vi "CheckClick.vi"(6 "Enum":enum16{"MouseClick", "DropDown"}(ring), 7 "Pad":string, 8 "error in (no error)":errorcluster, 10 "Coords":T1, 11 "EpiWrapper in":refnum<class "EpiWrapper.lvclass">) -> (0 "error out":errorcluster, 1 "OnPad?":bool, 2 "Selected?":bool, 3 "EpiWrapper out":refnum<class "EpiWrapper.lvclass">, 4 "Id":string)   [LabVIEW 2012, in "EpiWrapper.lvclass"]
uses:
  EpiWrapper.lvclass
  <vilib>/Utility/miscctls.llb/LVPoint32TypeDef.ctl
  EpiWrapper.lvclass/EpiWrapper.ctl
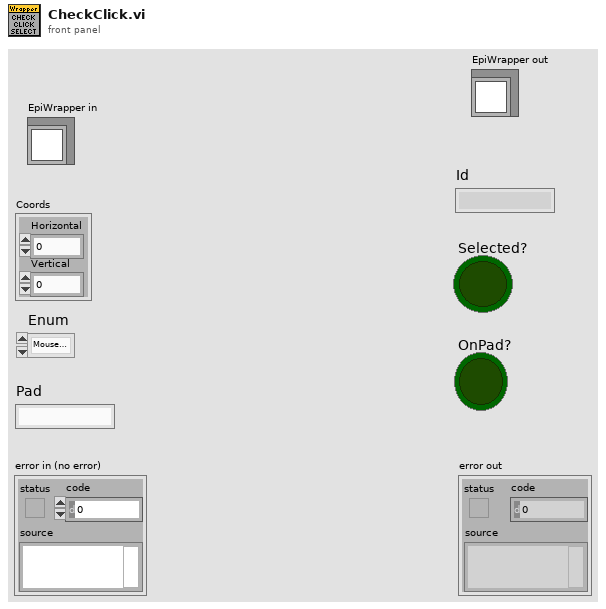
[diagram p1: front panel]
types:
  T1 = typedef "LVPoint32TypeDef.ctl" = cluster{"Horizontal":i32, "Vertical":i32}
  T2 = typedef "MapPOS.ctl" = cluster{"Coords":cluster{"Horizontal":sgl, "Vertical":sgl}, "radius":i32, "state":bool, "Id":string}[]
  T3 = typedef "SelectedPads.ctl" = T4[]
  T4 = typedef "Pad.ctl" = cluster{"Coords":cluster{"Horizontal":sgl, "Vertical":sgl}, "radius":i32, "Tested":bool, "Selected":bool, "Id":string}
  T5 = typedef "CurrentPad.ctl" = cluster{"Coords":cluster{"Horizontal":sgl, "Vertical":sgl}, "radius":i32, "Tested":bool, "Selected":bool, "Pad":string, "PadArea":T6}
  T6 = typedef "PadArea.ctl" = enum16{"A", "B", "C", "D", "L", "R", "T", "G"}
  T7 = typedef "MeasureControl.ctl" = cluster{"Graph":cluster{"Y":dbl[], "Y":dbl[]}[], "Pass":bool, "Fail":bool, "Measure":bool, "Wafer Area":T6, "TestData":T8, "Pad":string}
  T8 = typedef "TestData.ctl" = cluster{"20mA Data":T9, "50mA Data ":T9}
  T9 = typedef "Measurement.ctl" = cluster{"Area":string, "Pad":string, "Current,mA":dbl, "Power":dbl, "WL":dbl, "Voltage":dbl, "Knee Current":dbl, "Reverse":dbl}
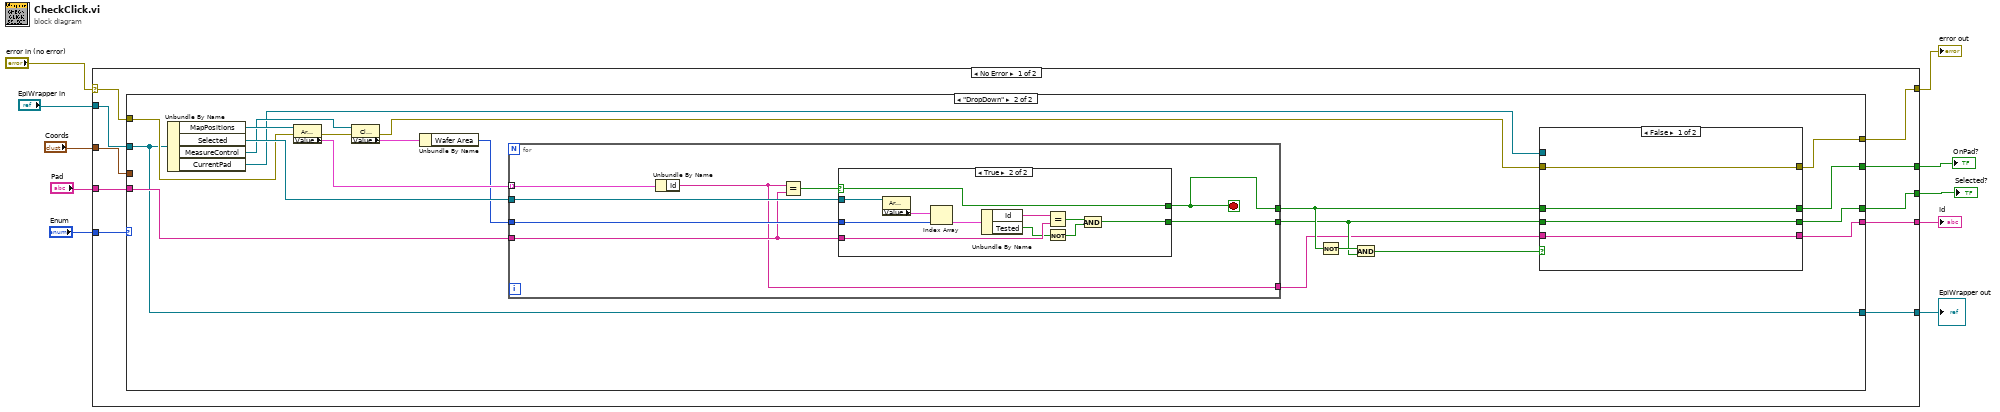
[diagram p0: block diagram]
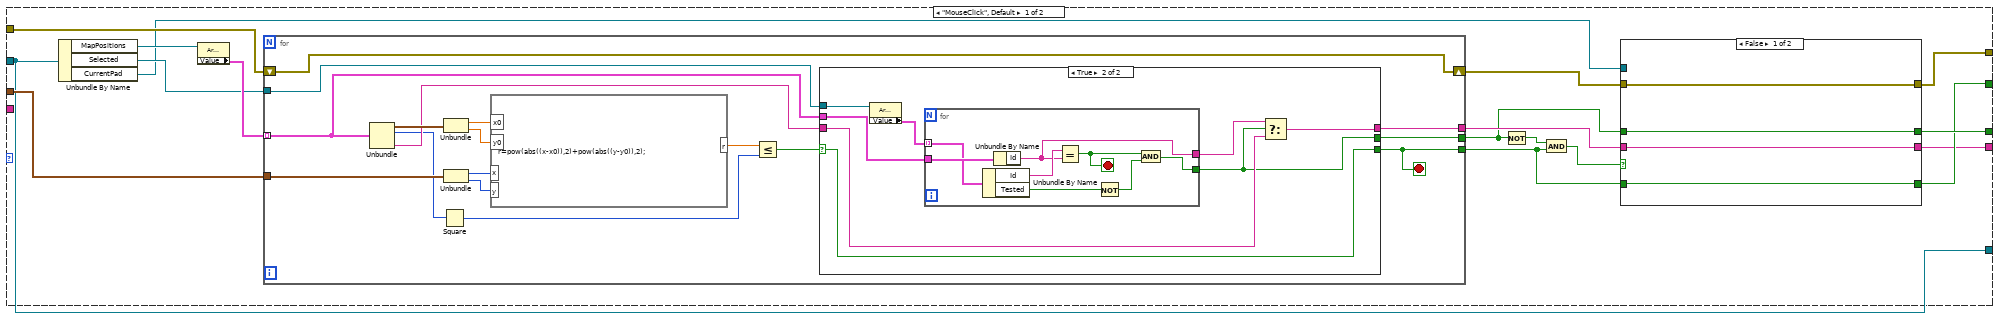
[diagram p2: hidden frame]
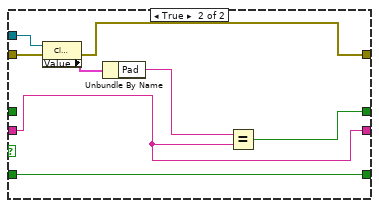
[diagram p3: hidden frame]
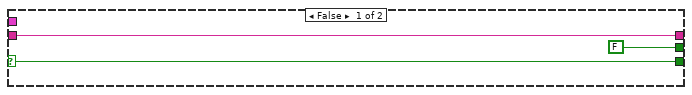
[diagram p4: hidden frame]
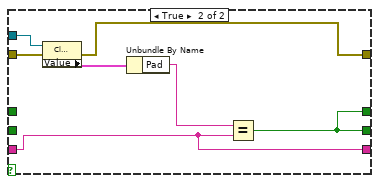
[diagram p5: hidden frame]
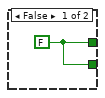
[diagram p6: hidden frame]
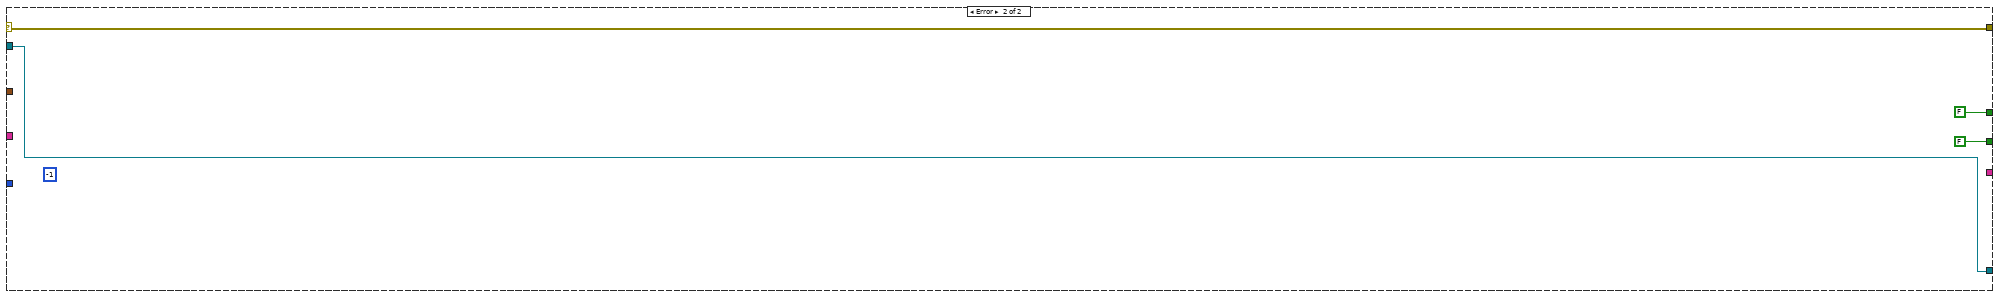
[diagram p7: hidden frame]
diagram:
  n1 = case shown="No Error" "error in (no error)" {
    selector: "error in (no error)" -> [w17 w141]
    tunnel: [w16 w141] -> w9
    tunnel: [w11 w140] -> w7
    tunnel: "EpiWrapper in" -> [w15 w140]
    tunnel: "Coords" -> [w20 _]
    tunnel: [w19 FALSE] -> w5
    tunnel: [w18 FALSE] -> w4
    tunnel: [w14 _] -> w3
    tunnel: "Enum" -> [w13 _]
    tunnel: "Pad" -> [w12 _]
    frame No Error {
      n2 = case shown="\"DropDown\"" w13 {
        tunnel: w20 -> [w35 _]
        tunnel: [w31 w92] -> w19
        tunnel: [w27 w91] -> w18
        tunnel: w17 -> [w33 w102]
        tunnel: [w23 w86] -> w16
        tunnel: w15 -> [w32 w99]
        tunnel: [w26 w88] -> w14
        tunnel: w12 -> [_ w104]
        tunnel: [w32 w99] -> w11
        frame "MouseClick", Default {
          n3 = Unbundle By Name(w32) -> ("MapPositions"=w37:refnum<vi>, "Selected"=w34:refnum<vi>, "CurrentPad"=w25:refnum<vi>)
          n4 = property class="Arr (strict)"(reference=w37) -> ("Value"=w36:T2)  [unwired: 1 in, 2 out]
          n5 = for {
            tunnel: w36 -> [w57] mode=indexing
            tunnel: w35 -> [w60]
            tunnel: w34 -> [w58]
            tunnel: [w56] -> w21
            tunnel: [w55] -> w22
            shift-right: [w54] -> w30
            shift-left: w33 -> [w54]
            tunnel: [w53] -> w24
            stop <- w55 stop-if-true
            n6 = Unbundle(w57) -> ("Coords"=w63:cluster{"Horizontal":sgl, "Vertical":sgl}, "radius"=w51:i32, "Id"=w52:string)  [unwired: 1 out]
            n7 = Square(x=w51) -> (x^2=w50:i32)
            n8 = Unbundle(w63) -> ("Horizontal"=w62:sgl, "Vertical"=w61:sgl)
            n9 = Unbundle(w60) -> ("Horizontal"=w66:i32, "Vertical"=w65:i32)
            n10 = formula code="r=pow(abs((x-x0)),2)+pow(abs((y-y0)),2);"("x0"=w62, "y0"=w61, "x"=w66, "y"=w65) -> ("r"=w64:dbl)
            n11 = Less Or Equal?(x=w64, y=w50) -> (x <= y?=w59:bool)
            n12 = case shown="True" w59 {
              selector: w59 -> [w69 w77]
              tunnel: [w69 w77] -> w55
              tunnel: w58 -> [_ w76]
              tunnel: w57 -> [_ w70]
              tunnel: [FALSE w72] -> w56
              tunnel: [w67 w73] -> w53
              tunnel: w52 -> [w67 w74]
              frame False {
              }
              frame True {
                n13 = property on="Property Node" class="Arr (strict)"(reference=w76) -> ("Value"=w71:T3)  [unwired: 1 in, 2 out]
                n14 = for {
                  tunnel: w70 -> [w83]
                  tunnel: [w81] -> w72
                  tunnel: [w84] -> w75
                  tunnel: w71 -> [w82] mode=indexing
                  stop <- w78 stop-if-true
                  n15 = Unbundle By Name(w82) -> ("Id"=w85:string, "Tested"=w80:bool)
                  n16 = Unbundle By Name(w83) -> ("Id"=w84:string)
                  n17 = Equal?(x=w85, y=w84) -> (x = y?=w78:bool)
                  n18 = Not(x=w80) -> (.not. x?=w79:bool)
                  n19 = And(x=w78, y=w79) -> (x .and. y?=w81:bool)
                }
                n20 = Select(t=w75, s=w72, f=w74) -> (s? t:f=w73:string)
              }
            }
          }
          n21 = Not(x=w21) -> (.not. x?=w28:bool)
          n22 = And(x=w28, y=w22) -> (x .and. y?=w29:bool)
          n23 = case shown="False" w29 {
            tunnel: [w39 w45] -> w31
            tunnel: w25 -> [_ w49]
            tunnel: w30 -> [w38 w48]
            tunnel: [w41 w44] -> w27
            tunnel: [w40 w42] -> w26
            tunnel: w22 -> [w41 w44]
            tunnel: w24 -> [w40 w42]
            tunnel: w21 -> [w39 _]
            tunnel: [w38 w46] -> w23
            frame False {
            }
            frame True {
              n24 = property class="Clust (strict)"(reference=w49, error in=w48) -> (error out=w46:errorcluster, "Value"=w47:T5)  [unwired: 1 out]
              n25 = Unbundle By Name(w47) -> ("Pad"=w43:string)
              n26 = Equal?(x=w43, y=w42) -> (x = y?=w45:bool)
            }
          }
        }
        frame "DropDown" {
          n27 = Unbundle By Name(w99) -> ("MapPositions"=w106:refnum<vi>, "Selected"=w103:refnum<vi>, "MeasureControl"=w101:refnum<vi>, "CurrentPad"=w94:refnum<vi>)
          n28 = property class="Arr (strict)"(reference=w106, error in=w102) -> (error out=w98:errorcluster, "Value"=w105:T2)  [unwired: 1 out]
          n29 = property class="Clust (strict)"(reference=w101, error in=w98) -> (error out=w93:errorcluster, "Value"=w97:T7)  [unwired: 1 out]
          n30 = Unbundle By Name(w97) -> ("Wafer Area"=w100:T6)
          n31 = for {
            tunnel: w105 -> [w118] mode=indexing
            tunnel: w104 -> [w121]
            tunnel: [w124] -> w90
            tunnel: w103 -> [w123]
            tunnel: w100 -> [w122]
            tunnel: [w120] -> w89
            tunnel: [w119] -> w87
            stop <- w124 stop-if-true
            n32 = Unbundle By Name(w118) -> ("Id"=w119:string)
            n33 = Equal?(x=w119, y=w121) -> (x = y?=w125:bool)
            n34 = case shown="True" w125 {
              selector: w125 -> [_ w137]
              tunnel: [w126 w137] -> w124
              tunnel: w123 -> [_ w136]
              tunnel: w122 -> [_ w134]
              tunnel: w121 -> [_ w132]
              tunnel: [w126 w127] -> w120
              frame False {
                w126 = FALSE
              }
              frame True {
                n35 = property class="Arr (strict)"(reference=w136) -> ("Value"=w135:T3)  [unwired: 1 in, 2 out]
                n36 = Index Array(array=w135, index=w134) -> (element=w131:T4)
                n37 = Unbundle By Name(w131) -> ("Id"=w133:string, "Tested"=w128:bool)
                n38 = Equal?(x=w133, y=w132) -> (x = y?=w130:bool)
                n39 = Not(x=w128) -> (.not. x?=w129:bool)
                n40 = And(x=w130, y=w129) -> (x .and. y?=w127:bool)
              }
            }
          }
          n41 = Not(x=w90) -> (.not. x?=w96:bool)
          n42 = And(x=w96, y=w89) -> (x .and. y?=w95:bool)
          n43 = case shown="False" w95 {
            tunnel: [w108 w114] -> w92
            tunnel: w94 -> [_ w117]
            tunnel: w93 -> [w107 w116]
            tunnel: [w110 w114] -> w91
            tunnel: [w109 w111] -> w88
            tunnel: w90 -> [w110 _]
            tunnel: w87 -> [w109 w111]
            tunnel: w89 -> [w108 _]
            tunnel: [w107 w115] -> w86
            frame False {
            }
            frame True {
              n44 = property class="Clust (strict)"(reference=w117, error in=w116) -> (error out=w115:errorcluster, "Value"=w113:T5)  [unwired: 1 out]
              n45 = Unbundle By Name(w113) -> ("Pad"=w112:string)
              n46 = Equal?(x=w112, y=w111) -> (x = y?=w114:bool)
            }
          }
        }
      }
    }
    frame Error {
      (unwired) -1 ("t")
    }
  }
  "error out" <- w9
  "EpiWrapper out" <- w7
  "Selected?" <- w5
  "OnPad?" <- w4
  "Id" <- w3
